vi "Configure Trigger Event LAN.vi"(0 "VISA resource name":refnum<visa-resource-name>, 1 "IP Address (0.0.0.0)":string="0.0.0.0", 2 "Simulate Line State(1 : High)":u16(ring)=1 items=["Low", "High"], 5 "Trigger Number (1)":i32=1, 7 "Trigger Mode (0: Falling and Rising Edge)":i32(ring) items=["Falling and Rising Edge", "Falling Edge", "Rising Edge", "Rising-A", "Rising-M", "Synchronous", "Synchronous-A", "Synchronous-M"], 9 "Event ID":string, 11 "error in (no error)":errorcluster, 12 "LAN Protocol (0: TCP)":i32(ring) items=["TCP", "UDP", "Multiple Case"]) -> (4 "VISA resource name out":refnum<visa-resource-name>, 15 "error out":errorcluster)   [LabVIEW 2019, in "Keithley 2600 Series.lvlib"]
doc: "Configures the events that cause LAN trigger to assert."
uses:
  Keithley 2600 Series.lvlib
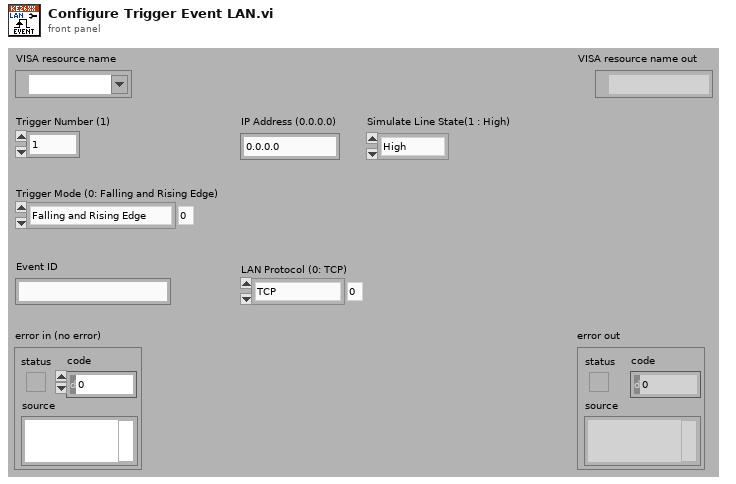
[diagram p1: front panel]
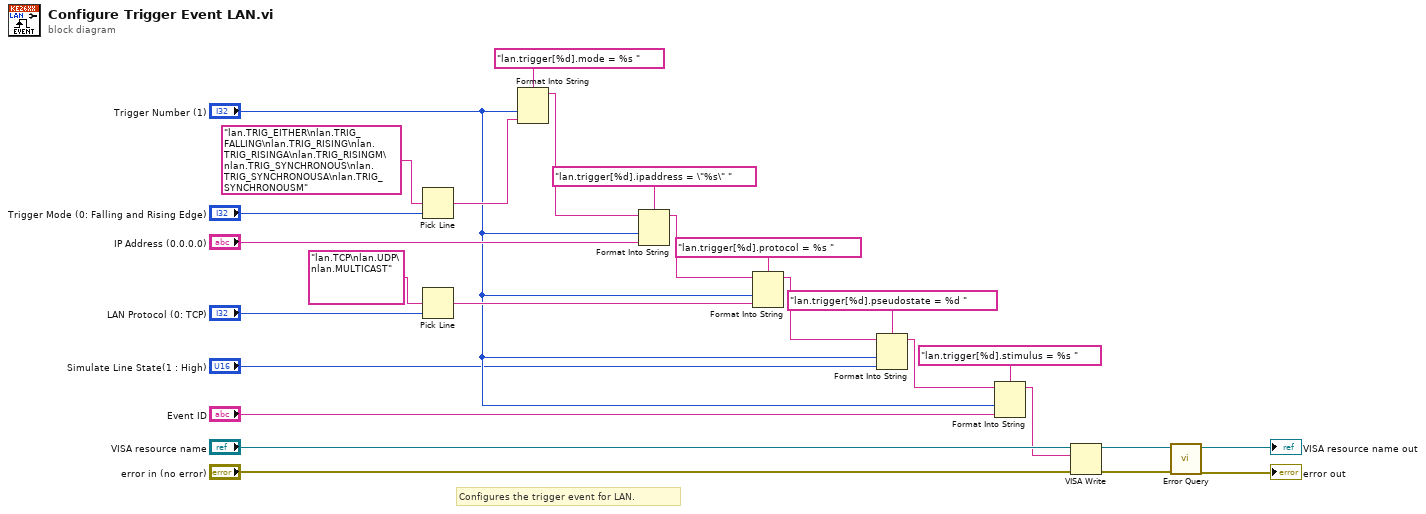
[diagram p0: block diagram]
diagram:
  # "Configures the trigger event for LAN."
  n1 = Pick Line(multi-line string="lan.TRIG_EITHER\nlan.TRIG_FALLING\nlan.TRIG_RISING\nlan.TRIG_RISINGA\nlan.TRIG_RISINGM\nlan.TRIG_SYNCHRONOUS\nlan.TRIG_SYNCHRONOUSA\nlan.TRIG_SYNCHRONOUSM", line index="Trigger Mode (0: Falling and Rising Edge)") -> (output string=w23:string)  [unwired: 1 in]
  n2 = Pick Line(multi-line string="lan.TCP\nlan.UDP\nlan.MULTICAST", line index="LAN Protocol (0: TCP)") -> (output string=w15:string)  [unwired: 1 in]
  n3 = Format Into String(format string="lan.trigger[%d].mode = %s ", "Trigger Number (1)", w23) -> (resulting string=w7:string)  [unwired: 2 in, 1 out]
  n4 = Format Into String(format string="lan.trigger[%d].ipaddress = \"%s\" ", initial string=w7, "Trigger Number (1)", "IP Address (0.0.0.0)") -> (resulting string=w6:string)  [unwired: 1 in, 1 out]
  n5 = Format Into String(format string="lan.trigger[%d].protocol = %s ", initial string=w6, "Trigger Number (1)", w15) -> (resulting string=w5:string)  [unwired: 1 in, 1 out]
  n6 = Format Into String(format string="lan.trigger[%d].pseudostate = %d ", initial string=w5, "Trigger Number (1)", "Simulate Line State(1 : High)") -> (resulting string=w4:string)  [unwired: 1 in, 1 out]
  n7 = Format Into String(format string="lan.trigger[%d].stimulus = %s ", initial string=w4, "Trigger Number (1)", "Event ID") -> (resulting string=w2:string)  [unwired: 1 in, 1 out]
  n8 = VISA Write(VISA resource name="VISA resource name", write buffer=w2, error in (no error)="error in (no error)") -> (VISA resource name out=w11:refnum<visa-resource-name>, error out=w10:errorcluster)  [unwired: 1 out]
  n9 = call "Error Query.vi"("error in (no error)"=w10, "VISA resource name"=w11) -> ("error out"=→"error out":errorcluster, "VISA resource name out"=→"VISA resource name out":refnum<visa-resource-name>)  [unwired: 6 in, 2 out]
